vi "换刀.vi"(8 "error in (no error)":errorcluster caption="错误输入（无错误）", 11 "钻削 输入":refnum<class "钻削.lvclass"> caption="DNL_LabVIEW Object in") -> (0 "error out":errorcluster caption="错误输出", 3 "钻削 输出":refnum<class "钻削.lvclass"> caption="DNL_LabVIEW Object out")   [LabVIEW 2011, in "钻削.lvclass"]
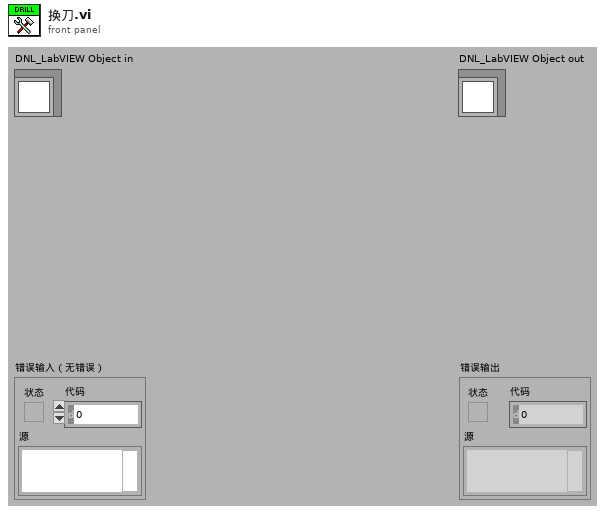
[diagram p1: front panel]
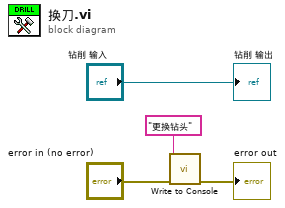
[diagram p0: block diagram]
diagram:
  n1 = call "Write to Console.vi"("error in (no error)"="error in (no error)", "Input"="更换钻头") -> ("error out"=→"error out":errorcluster)  [unwired: 9 in]
  "钻削 输出" <- "钻削 输入"
